vi "SetScreen.vi"(8 "Error In":errorcluster, 10 "Display Screen":T1, 11 "Keithley 2602 In":refnum<visa-resource-name>) -> (0 "Error Out":errorcluster, 3 "Keithley 2602 Out":refnum<visa-resource-name>)   [LabVIEW 2013, in "Keithley-2602.lvlib"]
uses:
  Keithley-2602.lvlib
  Controls/DisplayScreen.ctl
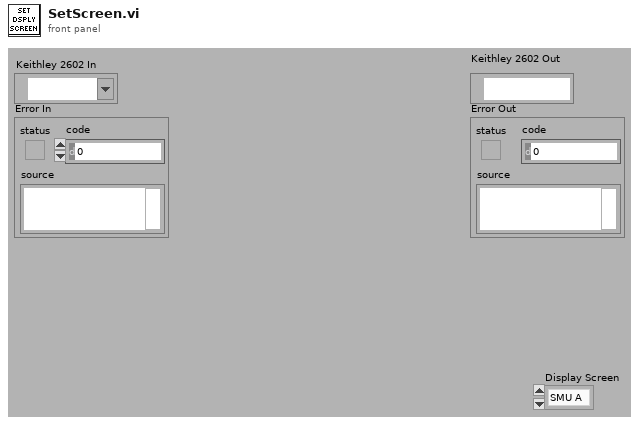
[diagram p1: front panel]
types:
  T1 = typedef "Keithley-2602.lvlib/DisplayScreen.ctl" = enum16{"SMU A", "SMU B", "Both", "User"}
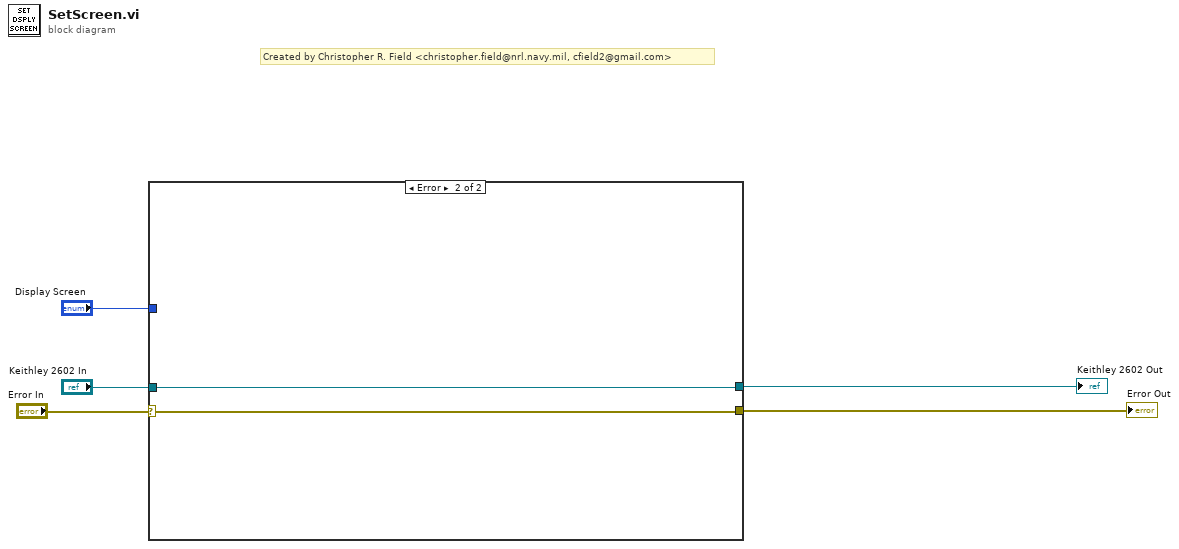
[diagram p0: block diagram]
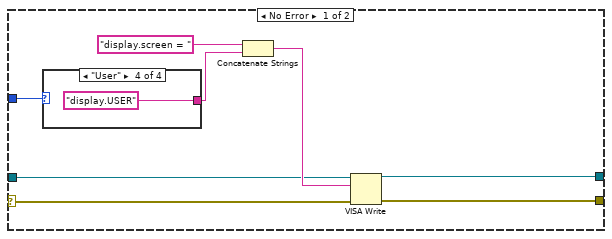
[diagram p2: hidden frame]
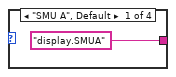
[diagram p3: hidden frame]
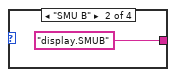
[diagram p4: hidden frame]
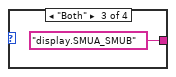
[diagram p5: hidden frame]
diagram:
  # "Created by Christopher R. Field <christopher.field@nrl.navy.mil, cfield2@gmail.com>"
  n1 = case shown="Error" "Error In" {
    selector: "Error In" -> [w6 w18]
    tunnel: "Keithley 2602 In" -> [w10 w19]
    tunnel: [w9 w19] -> w4
    tunnel: [w8 w18] -> w3
    tunnel: "Display Screen" -> [w7 _]
    frame No Error {
      n2 = case shown="\"User\"" w7 {
        tunnel: ["display.SMUA" "display.SMUB" "display.SMUA_SMUB" "display.USER"] -> w12
        frame "SMU A", Default {
        }
        frame "SMU B" {
        }
        frame "Both" {
        }
        frame "User" {
        }
      }
      n3 = Concatenate Strings("display.screen = ", w12) -> (w11:string)
      n4 = VISA Write(VISA resource name=w10, write buffer=w11, error in (no error)=w6) -> (VISA resource name out=w9:refnum<visa-resource-name>, error out=w8:errorcluster)  [unwired: 1 out]
    }
    frame Error {
    }
  }
  "Keithley 2602 Out" <- w4
  "Error Out" <- w3
